vi "Scale Cell Voltage.vi"(11 "Numeric in":u8) -> (3 "Numeric out":dbl)   [LabVIEW 2015]
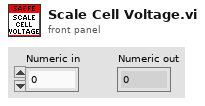
[diagram p1: front panel]
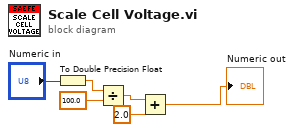
[diagram p0: block diagram]
diagram:
  n1 = To Double Precision Float(number="Numeric in") -> (double precision float=w5:dbl)
  n2 = Divide(x=w5, y=100.0) -> (x/y=w3:dbl)
  n3 = Add(x=w3, y=2.0) -> (x+y=→"Numeric out":dbl)
